vi "YAG AOM Pulse Control.vi"() -> ()   [LabVIEW 2012]
doc: "Shows how to configure then create an arbitrary waveform."
uses:
  Trap Frequency AFG Control/Public/Agilent 33XXX Series.lvlib
panel:
  in  "Start Time":i32=1
  in  "Step Voltage":dbl
  in  "Step Time":i32=15998
  in  "Initial Voltage":dbl=7.78
  out "Offset":dbl
  out "Amplitude":dbl
  out "Frequency":dbl=0.4838
  in  "Trigger Source (0: Internal)":u16(ring)=1 items=["Internal", "External", "Software (bus)"]
  in  "Enable Burst":bool=TRUE
  in  "Burst Mode (0: Triggered)":u16(ring) items=["Triggered", "Gated"]
  out "Simulated WaveForm":dbl[](graph)
  out "Total Time  (<16000)":i32
  in  "VISA resource name":refnum<visa-resource-name>="GPIB0::2::INSTR"
  in  "Arbitrary Waveform Name":string="ARB1"
  # "Read me: (Very Important!!!!!!!!!)\n1. This Labview is used to control the IPG laser output power, When you edit this programme make sure the IPG laser is off.\n2. follow the steps, First is the visa address setting; Second is the pulse edit; Third is the output checking; Forth is the trigger set .\n3. The maximum input voltage is 10V, the minmum value is 1V. The total input time must smaller than 16000ms and larger than 8 ms."
  # "IPG Laser Pulse Controller\n                             ----- FORT trap depth control"
  # "Setp 1"
  # "Setp 3"
  # "Setp 2"
  # "(  )"
  # "Time (  )"
  # "Voltage (V)"
  # "(Hz)"
  # "(V)"
  # "(V)"
  # "Setp 4"
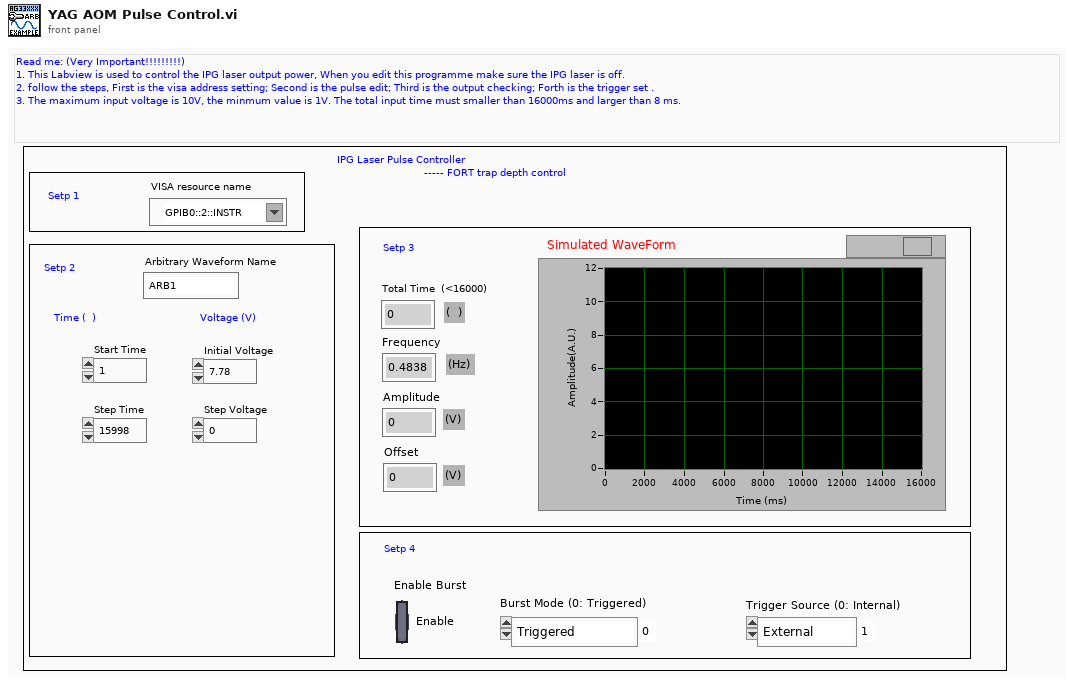
[diagram p1: front panel]
types:
  T1 = cluster{"Baud Rate":u32, "Parity":u16, "Data Bits":u16, "Flow Control":u16}
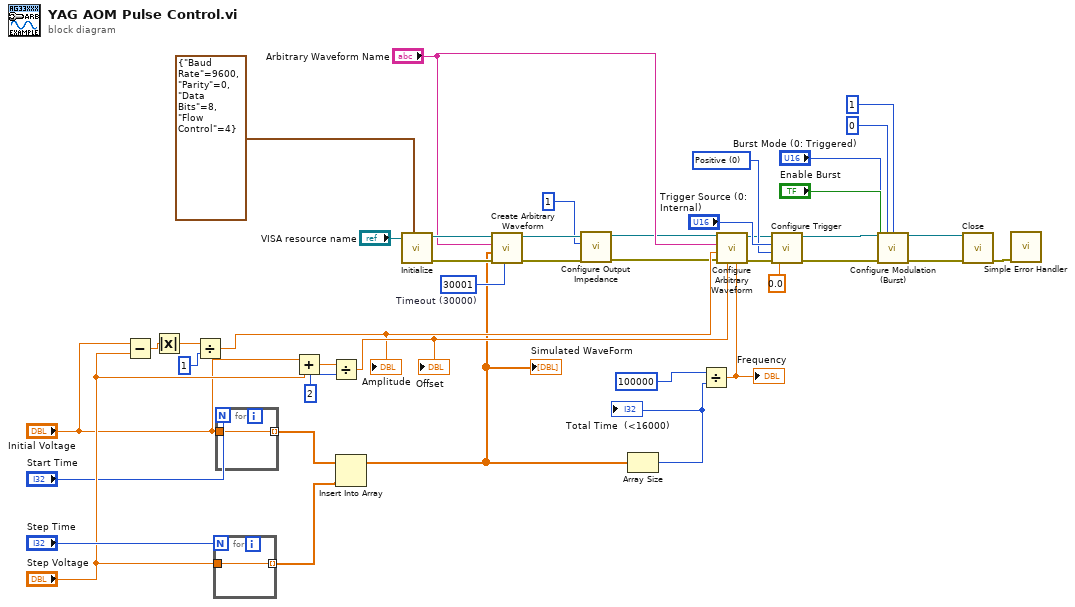
[diagram p0: block diagram]
diagram:
  w38 = u16 0 items=["Positive", "Negative"] ("Slope (0: Positive)")
  w23 = u32 30001  # Timeout (30000)
  n1 = Subtract(x="Initial Voltage", y="Step Voltage") -> (x-y=w17:dbl)
  n2 = Absolute Value(x=w17) -> (abs(x)=w16:dbl)
  n3 = Divide(x=w16, y=1) -> (x/y=w15:dbl)
  "Amplitude" <- w15
  n4 = for {
    N: "Step Time" -> [_]
    tunnel: [w43] -> w9 mode=indexing
    tunnel: "Step Voltage" -> [w43]
  }
  n5 = for {
    N: "Start Time" -> [_]
    tunnel: [w44] -> w11 mode=indexing
    tunnel: "Initial Voltage" -> [w44]
  }
  n6 = Add(x="Initial Voltage", y="Step Voltage") -> (x+y=w21:dbl)
  n7 = Divide(x=w21, y=2) -> (x/y=w19:dbl)
  "Offset" <- w19
  n8 = Insert Into Array(array=w11, new element=w9) -> (w14:dbl[])  [unwired: 1 in]
  "Simulated WaveForm" <- w14
  n9 = call "Initialize.vi"("Serial Configuration"=T1 {"Baud Rate"=9600, "Parity"=0, "Data Bits"=8, "Flow Control"=4}, "VISA resource name"="VISA resource name") -> ("error out"=w24:errorcluster, "VISA resource name out"=w25:refnum<visa-resource-name>)  [unwired: 8 in]
  n10 = call "Create Arbitrary Waveform.vi"("Timeout (10000)"=w23, "error in (no error)"=w24, "Arbitrary Waveform Data"=w14, "Arbitrary Waveform Name (\"ARB1\")"="Arbitrary Waveform Name", "VISA resource name"=w25) -> ("error out"=w3:errorcluster, "VISA resource name out"=w5:refnum<visa-resource-name>)  [unwired: 5 in]
  n11 = call "Configure Output Impedance.vi"("error in (no error)"=w3, "Impedance (0: 50 Ohms)"=1, "VISA resource name"=w5) -> ("error out"=w2:errorcluster, "VISA resource name out"=w4:refnum<visa-resource-name>)  [unwired: 7 in]
  n12 = Array Size(array=w14) -> (size(s)=w26:i32)
  "Total Time  (<16000)" <- w26
  n13 = Divide(x=100000, y=w26) -> (x/y=w27:dbl)
  "Frequency" <- w27
  n14 = call "Configure Arbitrary Waveform.vi"("Frequency (1000 Hz)"=w27, "Offset (0.00 V)"=w19, "error in (no error)"=w2, "Gain (1.0)"=w15, "Arbitrary Waveform Name (\"ARB1\")"="Arbitrary Waveform Name", "VISA resource name"=w4) -> ("error out"=w36:errorcluster, "VISA resource name out"=w37:refnum<visa-resource-name>)  [unwired: 4 in]
  n15 = call "Configure Trigger.vi"("Delay (0.0 s)"=0.0, "error in (no error)"=w36, "Slope (0: Positive)"=w38, "Trigger Source (0: Internal)"="Trigger Source (0: Internal)", "VISA resource name"=w37) -> ("error out"=w34:errorcluster, "VISA resource name out"=w35:refnum<visa-resource-name>)  [unwired: 5 in]
  n16 = call "Configure Modulation (Burst).vi"("VISA resource name"=w35, "Burst Phase (0 deg)"=0, "Burst Count (1)"=1, "Enable Burst Modulation (T: Enable)"="Enable Burst", "Burst Modulation Mode (0: Triggered)"="Burst Mode (0: Triggered)", "error in (no error)"=w34) -> ("VISA resource name out"=w13:refnum<visa-resource-name>, "error out"=w12:errorcluster)  [unwired: 8 in]
  n17 = call "Close.vi"("error in (no error)"=w12, "VISA resource name"=w13) -> ("error out"=w42:errorcluster)  [unwired: 9 in]
  n18 = call <vilib>:"Simple Error Handler.vi"("error in (no error)"=w42) -> ()  [unwired: 4 in, 5 out]
